vi "Relationship Check.vi"(5 "TestRef":refnum<vi>, 9 "reference in":refnum<vi>) -> (0 "Is TestRef":bool, 3 "Is Child of TestRef":bool)   [LabVIEW 2020, in "CSM-Helper.lvclass"]
uses:
  CSM-Helper.lvclass
  CSM-Helper.lvclass/CSM-Helper.ctl
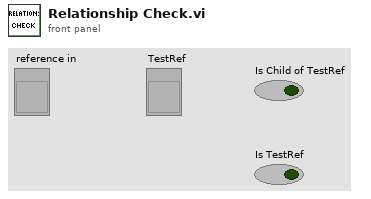
[diagram p1: front panel]
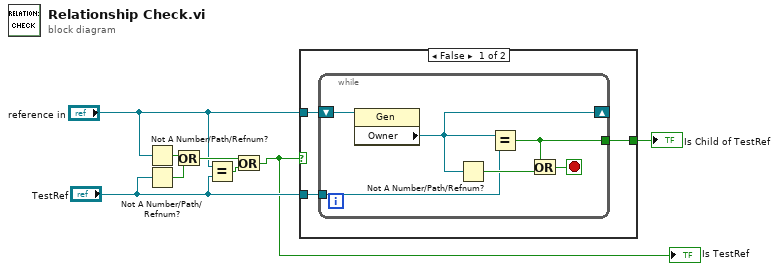
[diagram p0: block diagram]
diagram:
  n1 = Not A Number/Path/Refnum?(number/path/refnum="reference in") -> (NaN/Path/Refnum?=w6:bool)
  n2 = Not A Number/Path/Refnum?(number/path/refnum="TestRef") -> (NaN/Path/Refnum?=w7:bool)
  n3 = Or(x=w6, y=w7) -> (x .or. y?=w8:bool)
  n4 = Equal?(x="reference in", y="TestRef") -> (x = y?=w4:bool)
  n5 = Or(x=w8, y=w4) -> (x .or. y?=w1:bool)
  "Is TestRef" <- w1
  n6 = case shown="False" w1 {
    tunnel: [w11 _] -> w5
    tunnel: "reference in" -> [w10 _]
    tunnel: "TestRef" -> [w9 _]
    frame False {
      n7 = while {
        tunnel: w9 -> [w12]
        tunnel: [w14] -> w11
        shift-right: [w13] -> _
        shift-left: w10 -> [w17]
        stop <- w16 stop-if-true
        n8 = property class="Gen"(reference=w17) -> ("Owner"=w13:refnum<vi>)  [unwired: 1 in, 2 out]
        n9 = Not A Number/Path/Refnum?(number/path/refnum=w13) -> (NaN/Path/Refnum?=w15:bool)
        n10 = Equal?(x=w13, y=w12) -> (x = y?=w14:bool)
        n11 = Or(x=w14, y=w15) -> (x .or. y?=w16:bool)
      }
    }
    frame True {
    }
  }
  "Is Child of TestRef" <- w5
